vi "Init from Ref.vi"(10 "Cell Ref":refnum<k24>, 11 "Cell in":refnum<class "Cell.lvclass">) -> (3 "Cell out":refnum<class "Cell.lvclass">)   [LabVIEW 2024, in "SourceGrid.lvlib" / "Cell.lvclass"]
uses:
  Cell.lvclass
  Cell.lvclass/Cell.ctl
  D:/git/Sourcegrid-LabVIEW/dll/SourceGrid.dll
  dll/SourceGrid.dll
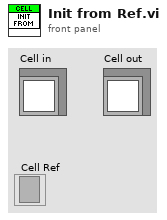
[diagram p1: front panel]
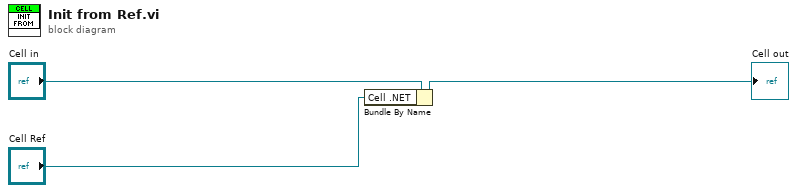
[diagram p0: block diagram]
diagram:
  n1 = Bundle By Name(cluster="Cell in", "Cell .NET"="Cell Ref") -> (→"Cell out":refnum<class "Cell.lvclass">)
